vi "SequenceDemo.vi"(8 "error in (no error)":errorcluster, 10 "Sequence Paras":T1 {"End position" format="%.2f"; "Start position" format="%.2f"}, 11 "lLSID":i32) -> (0 "error out":errorcluster)   [LabVIEW 2011]
uses:
  SequenceParam.ctl
  <userlib>/Tango_DLL/Tango_DLL.lvlib
panel:
  out "End position":dbl[](array[numeric]) format="%.2f"
  out "Start position":dbl[](array[numeric]) format="%.2f"
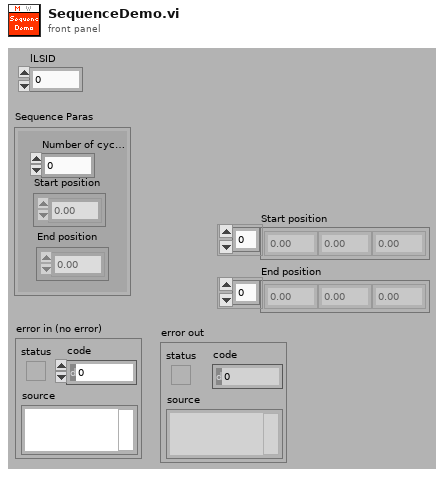
[diagram p1: front panel]
types:
  T1 = typedef "SequenceParam.ctl" = cluster{"Number of cycles":i32, "Start position":dbl[], "End position":dbl[]}
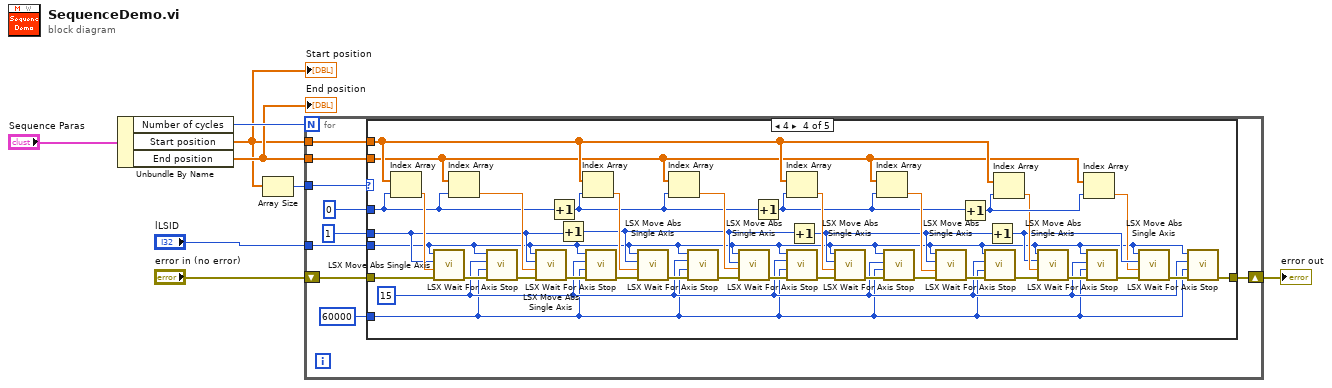
[diagram p0: block diagram]
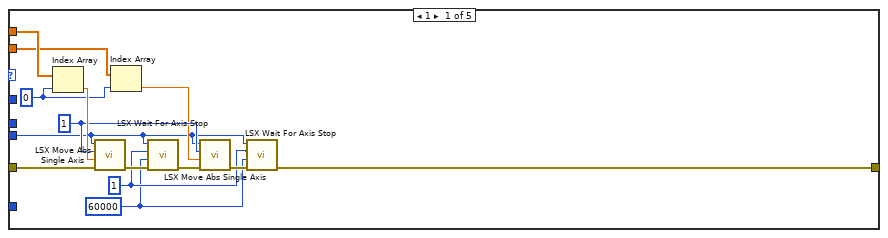
[diagram p2: hidden frame]
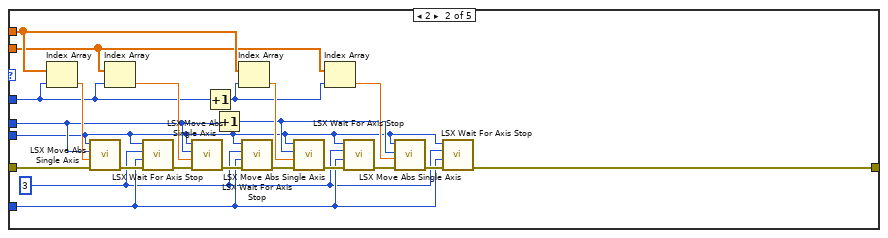
[diagram p3: hidden frame]
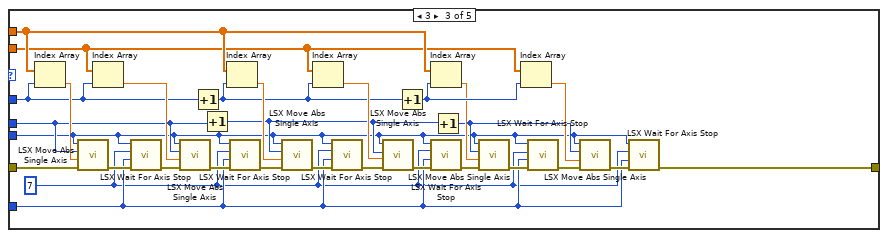
[diagram p4: hidden frame]
diagram:
  n1 = Unbundle By Name("Sequence Paras") -> ("Number of cycles"=w6:i32, "Start position"=w2:dbl[], "End position"=w5:dbl[])
  "Start position" <- w2
  "End position" <- w5
  n2 = Array Size(array=w2) -> (size(s)=w1:i32)
  n3 = for {
    N: w6 -> [_]
    shift-right: [w12] -> w7
    shift-left: "error in (no error)" -> [w17]
    tunnel: w2 -> [w15]
    tunnel: w5 -> [w13]
    tunnel: "lLSID" -> [w16]
    tunnel: w1 -> [w14]
    n4 = case shown="4" w14 {
      tunnel: w17 -> [w28 w53 w72 w102 w122]
      tunnel: w16 -> [w18 w32 w54 w84 _]
      tunnel: w15 -> [w29 w47 w68 w98 _]
      tunnel: w13 -> [w24 w42 w67 w97 _]
      tunnel: [w19 w37 w56 w91 w122] -> w12
      tunnel: 0 ("Index") -> [_ w36 w70 w100 _]
      tunnel: 1 -> [_ w35 w71 w101 _]
      tunnel: 60000 ("lATimeoutValue") -> [_ w34 w57 w85 _]
      frame 1 {
        w26 = 1 ("lAxis")
        w25 = 0 ("Index")
        w20 = 60000 ("lATimeoutValue")
        w21 = 1 ("lAFlags")
        n5 = Index Array(array=w29, index=w25) -> (element=w31:dbl)
        n6 = call <userlib>:"LSX Move Abs Single Axis.vi"("error in (no error)"=w28, "dValue"=w31, "lAxis"=w26, "lLSID"=w18) -> ("error out"=w30:errorcluster)  [unwired: 6 in, 1 out]
        n7 = Index Array(array=w24, index=w25) -> (element=w23:dbl)
        n8 = call <userlib>:"LSX Wait For Axis Stop.vi"("error in (no error)"=w30, "lATimeoutValue"=w20, "lAFlags"=w21, "lLSID"=w18) -> ("error out"=w27:errorcluster)  [unwired: 5 in, 2 out]
        n9 = call <userlib>:"LSX Move Abs Single Axis.vi"("error in (no error)"=w27, "dValue"=w23, "lAxis"=w26, "lLSID"=w18) -> ("error out"=w22:errorcluster)  [unwired: 6 in, 1 out]
        n10 = call <userlib>:"LSX Wait For Axis Stop.vi"("error in (no error)"=w22, "lATimeoutValue"=w20, "lAFlags"=w21, "lLSID"=w18) -> ("error out"=w19:errorcluster)  [unwired: 5 in, 2 out]
      }
      frame 2 {
        w33 = 3 ("lAFlags")
        n11 = Index Array(array=w47, index=w36) -> (element=w52:dbl)
        n12 = call <userlib>:"LSX Move Abs Single Axis.vi"("error in (no error)"=w53, "dValue"=w52, "lAxis"=w35, "lLSID"=w32) -> ("error out"=w51:errorcluster)  [unwired: 6 in, 1 out]
        n13 = Index Array(array=w42, index=w36) -> (element=w49:dbl)
        n14 = call <userlib>:"LSX Wait For Axis Stop.vi"("error in (no error)"=w51, "lATimeoutValue"=w34, "lAFlags"=w33, "lLSID"=w32) -> ("error out"=w50:errorcluster)  [unwired: 5 in, 2 out]
        n15 = call <userlib>:"LSX Move Abs Single Axis.vi"("error in (no error)"=w50, "dValue"=w49, "lAxis"=w35, "lLSID"=w32) -> ("error out"=w48:errorcluster)  [unwired: 6 in, 1 out]
        n16 = Increment(x=w36) -> (x+1=w41:i32)
        n17 = Increment(x=w35) -> (x+1=w39:i32)
        n18 = Index Array(array=w47, index=w41) -> (element=w45:dbl)
        n19 = call <userlib>:"LSX Wait For Axis Stop.vi"("error in (no error)"=w48, "lATimeoutValue"=w34, "lAFlags"=w33, "lLSID"=w32) -> ("error out"=w46:errorcluster)  [unwired: 5 in, 2 out]
        n20 = call <userlib>:"LSX Move Abs Single Axis.vi"("error in (no error)"=w46, "dValue"=w45, "lAxis"=w39, "lLSID"=w32) -> ("error out"=w44:errorcluster)  [unwired: 6 in, 1 out]
        n21 = Index Array(array=w42, index=w41) -> (element=w40:dbl)
        n22 = call <userlib>:"LSX Wait For Axis Stop.vi"("error in (no error)"=w44, "lATimeoutValue"=w34, "lAFlags"=w33, "lLSID"=w32) -> ("error out"=w43:errorcluster)  [unwired: 5 in, 2 out]
        n23 = call <userlib>:"LSX Move Abs Single Axis.vi"("error in (no error)"=w43, "dValue"=w40, "lAxis"=w39, "lLSID"=w32) -> ("error out"=w38:errorcluster)  [unwired: 6 in, 1 out]
        n24 = call <userlib>:"LSX Wait For Axis Stop.vi"("error in (no error)"=w38, "lATimeoutValue"=w34, "lAFlags"=w33, "lLSID"=w32) -> ("error out"=w37:errorcluster)  [unwired: 5 in, 2 out]
      }
      frame 3 {
        w55 = 7 ("lAFlags")
        n25 = Index Array(array=w68, index=w70) -> (element=w83:dbl)
        n26 = call <userlib>:"LSX Move Abs Single Axis.vi"("error in (no error)"=w72, "dValue"=w83, "lAxis"=w71, "lLSID"=w54) -> ("error out"=w82:errorcluster)  [unwired: 6 in, 1 out]
        n27 = Index Array(array=w67, index=w70) -> (element=w80:dbl)
        n28 = call <userlib>:"LSX Wait For Axis Stop.vi"("error in (no error)"=w82, "lATimeoutValue"=w57, "lAFlags"=w55, "lLSID"=w54) -> ("error out"=w81:errorcluster)  [unwired: 5 in, 2 out]
        n29 = call <userlib>:"LSX Move Abs Single Axis.vi"("error in (no error)"=w81, "dValue"=w80, "lAxis"=w71, "lLSID"=w54) -> ("error out"=w79:errorcluster)  [unwired: 6 in, 1 out]
        n30 = Increment(x=w70) -> (x+1=w66:i32)
        n31 = Increment(x=w71) -> (x+1=w62:i32)
        n32 = Index Array(array=w68, index=w66) -> (element=w77:dbl)
        n33 = call <userlib>:"LSX Wait For Axis Stop.vi"("error in (no error)"=w79, "lATimeoutValue"=w57, "lAFlags"=w55, "lLSID"=w54) -> ("error out"=w78:errorcluster)  [unwired: 5 in, 2 out]
        n34 = call <userlib>:"LSX Move Abs Single Axis.vi"("error in (no error)"=w78, "dValue"=w77, "lAxis"=w62, "lLSID"=w54) -> ("error out"=w76:errorcluster)  [unwired: 6 in, 1 out]
        n35 = Index Array(array=w67, index=w66) -> (element=w74:dbl)
        n36 = call <userlib>:"LSX Wait For Axis Stop.vi"("error in (no error)"=w76, "lATimeoutValue"=w57, "lAFlags"=w55, "lLSID"=w54) -> ("error out"=w75:errorcluster)  [unwired: 5 in, 2 out]
        n37 = call <userlib>:"LSX Move Abs Single Axis.vi"("error in (no error)"=w75, "dValue"=w74, "lAxis"=w62, "lLSID"=w54) -> ("error out"=w73:errorcluster)  [unwired: 6 in, 1 out]
        n38 = Increment(x=w66) -> (x+1=w69:i32)
        n39 = Index Array(array=w68, index=w69) -> (element=w63:dbl)
        n40 = call <userlib>:"LSX Wait For Axis Stop.vi"("error in (no error)"=w73, "lATimeoutValue"=w57, "lAFlags"=w55, "lLSID"=w54) -> ("error out"=w64:errorcluster)  [unwired: 5 in, 2 out]
        n41 = Increment(x=w62) -> (x+1=w58:i32)
        n42 = call <userlib>:"LSX Move Abs Single Axis.vi"("error in (no error)"=w64, "dValue"=w63, "lAxis"=w58, "lLSID"=w54) -> ("error out"=w65:errorcluster)  [unwired: 6 in, 1 out]
        n43 = Index Array(array=w67, index=w69) -> (element=w59:dbl)
        n44 = call <userlib>:"LSX Wait For Axis Stop.vi"("error in (no error)"=w65, "lATimeoutValue"=w57, "lAFlags"=w55, "lLSID"=w54) -> ("error out"=w60:errorcluster)  [unwired: 5 in, 2 out]
        n45 = call <userlib>:"LSX Move Abs Single Axis.vi"("error in (no error)"=w60, "dValue"=w59, "lAxis"=w58, "lLSID"=w54) -> ("error out"=w61:errorcluster)  [unwired: 6 in, 1 out]
        n46 = call <userlib>:"LSX Wait For Axis Stop.vi"("error in (no error)"=w61, "lATimeoutValue"=w57, "lAFlags"=w55, "lLSID"=w54) -> ("error out"=w56:errorcluster)  [unwired: 5 in, 2 out]
      }
      frame 4 {
        w86 = 15 ("lAFlags")
        n47 = Index Array(array=w98, index=w100) -> (element=w121:dbl)
        n48 = call <userlib>:"LSX Move Abs Single Axis.vi"("error in (no error)"=w102, "dValue"=w121, "lAxis"=w101, "lLSID"=w84) -> ("error out"=w120:errorcluster)  [unwired: 6 in, 1 out]
        n49 = Index Array(array=w97, index=w100) -> (element=w118:dbl)
        n50 = call <userlib>:"LSX Wait For Axis Stop.vi"("error in (no error)"=w120, "lATimeoutValue"=w85, "lAFlags"=w86, "lLSID"=w84) -> ("error out"=w119:errorcluster)  [unwired: 5 in, 2 out]
        n51 = call <userlib>:"LSX Move Abs Single Axis.vi"("error in (no error)"=w119, "dValue"=w118, "lAxis"=w101, "lLSID"=w84) -> ("error out"=w117:errorcluster)  [unwired: 6 in, 1 out]
        n52 = Increment(x=w100) -> (x+1=w110:i32)
        n53 = Increment(x=w101) -> (x+1=w106:i32)
        n54 = Index Array(array=w98, index=w110) -> (element=w115:dbl)
        n55 = call <userlib>:"LSX Wait For Axis Stop.vi"("error in (no error)"=w117, "lATimeoutValue"=w85, "lAFlags"=w86, "lLSID"=w84) -> ("error out"=w116:errorcluster)  [unwired: 5 in, 2 out]
        n56 = call <userlib>:"LSX Move Abs Single Axis.vi"("error in (no error)"=w116, "dValue"=w115, "lAxis"=w106, "lLSID"=w84) -> ("error out"=w114:errorcluster)  [unwired: 6 in, 1 out]
        n57 = Index Array(array=w97, index=w110) -> (element=w112:dbl)
        n58 = call <userlib>:"LSX Wait For Axis Stop.vi"("error in (no error)"=w114, "lATimeoutValue"=w85, "lAFlags"=w86, "lLSID"=w84) -> ("error out"=w113:errorcluster)  [unwired: 5 in, 2 out]
        n59 = call <userlib>:"LSX Move Abs Single Axis.vi"("error in (no error)"=w113, "dValue"=w112, "lAxis"=w106, "lLSID"=w84) -> ("error out"=w111:errorcluster)  [unwired: 6 in, 1 out]
        n60 = Increment(x=w110) -> (x+1=w96:i32)
        n61 = Index Array(array=w98, index=w96) -> (element=w107:dbl)
        n62 = call <userlib>:"LSX Wait For Axis Stop.vi"("error in (no error)"=w111, "lATimeoutValue"=w85, "lAFlags"=w86, "lLSID"=w84) -> ("error out"=w108:errorcluster)  [unwired: 5 in, 2 out]
        n63 = Increment(x=w106) -> (x+1=w95:i32)
        n64 = call <userlib>:"LSX Move Abs Single Axis.vi"("error in (no error)"=w108, "dValue"=w107, "lAxis"=w95, "lLSID"=w84) -> ("error out"=w109:errorcluster)  [unwired: 6 in, 1 out]
        n65 = Index Array(array=w97, index=w96) -> (element=w103:dbl)
        n66 = call <userlib>:"LSX Wait For Axis Stop.vi"("error in (no error)"=w109, "lATimeoutValue"=w85, "lAFlags"=w86, "lLSID"=w84) -> ("error out"=w104:errorcluster)  [unwired: 5 in, 2 out]
        n67 = call <userlib>:"LSX Move Abs Single Axis.vi"("error in (no error)"=w104, "dValue"=w103, "lAxis"=w95, "lLSID"=w84) -> ("error out"=w105:errorcluster)  [unwired: 6 in, 1 out]
        n68 = Increment(x=w96) -> (x+1=w99:i32)
        n69 = call <userlib>:"LSX Wait For Axis Stop.vi"("error in (no error)"=w105, "lATimeoutValue"=w85, "lAFlags"=w86, "lLSID"=w84) -> ("error out"=w89:errorcluster)  [unwired: 5 in, 2 out]
        n70 = Increment(x=w95) -> (x+1=w88:i32)
        n71 = Index Array(array=w98, index=w99) -> (element=w90:dbl)
        n72 = call <userlib>:"LSX Move Abs Single Axis.vi"("error in (no error)"=w89, "dValue"=w90, "lAxis"=w88, "lLSID"=w84) -> ("error out"=w92:errorcluster)  [unwired: 6 in, 1 out]
        n73 = Index Array(array=w97, index=w99) -> (element=w87:dbl)
        n74 = call <userlib>:"LSX Wait For Axis Stop.vi"("error in (no error)"=w92, "lATimeoutValue"=w85, "lAFlags"=w86, "lLSID"=w84) -> ("error out"=w94:errorcluster)  [unwired: 5 in, 2 out]
        n75 = call <userlib>:"LSX Move Abs Single Axis.vi"("error in (no error)"=w94, "dValue"=w87, "lAxis"=w88, "lLSID"=w84) -> ("error out"=w93:errorcluster)  [unwired: 6 in, 1 out]
        n76 = call <userlib>:"LSX Wait For Axis Stop.vi"("error in (no error)"=w93, "lATimeoutValue"=w85, "lAFlags"=w86, "lLSID"=w84) -> ("error out"=w91:errorcluster)  [unwired: 5 in, 2 out]
      }
      frame Default {
      }
    }
  }
  "error out" <- w7
